vi "Express Waveform Components.vi"(8 "error in (no error)":errorcluster, 11 "Waveform":waveform(dbl)) -> (0 "error out":errorcluster, 1 "Express Waveform Attributes":T1 {"Timestamp" format="%<%X\n%x>T"; "Start Timestamp" format="%<%X\n%x>T"}, 2 "Signal Components":cluster{"X0":dbl, "dX":dbl, "Y":dbl[]} {"Y" format="%0.2f"; "dX" format="%0.6f"; "X0" format="%0.6f"}, 3 "Waveform":waveform(dbl))   [LabVIEW 2020]
uses:
  <vilib>/express/express shared/transition.llb/ex_WaveformAttribs.ctl
panel:
  in  "signal":cluster{"X0":dbl, "dX":dbl, "Y":dbl[]} {"X0" format="%.6f"; "dX" format="%.6f"; "Y" format="%0.2p"}
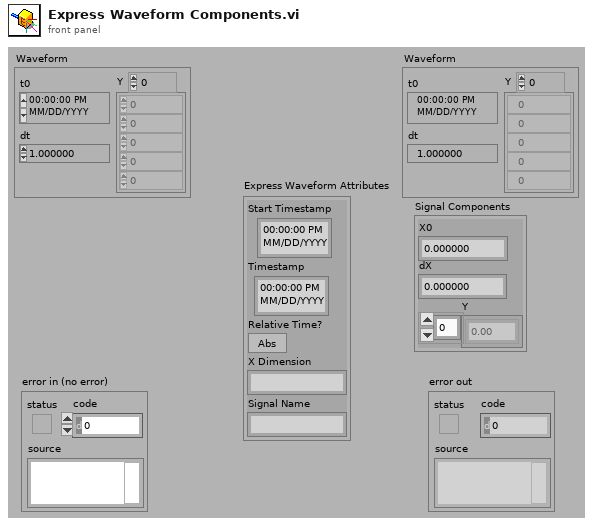
[diagram p1: front panel]
types:
  T1 = typedef "ex_WaveformAttribs.ctl" = cluster{"Start Timestamp":timestamp, "Timestamp":timestamp, "Relative Time?":bool, "X Dimension":string, "Signal Name":string}
  T2 = cluster{"Start Timestamp":timestamp, "Timestamp":timestamp, "Relative Time?":bool, "X Dimension":string, "Signal Name":string}[]
  T3 = cluster{"Start Timestamp":timestamp, "Timestamp":timestamp, "Relative Time?":bool, "X Dimension":string, "Signal Name":string}
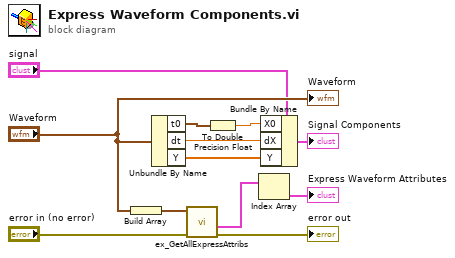
[diagram p0: block diagram]
diagram:
  n1 = Build Array("Waveform") -> (w6:waveform(dbl)[])
  n2 = Unbundle By Name("Waveform") -> ("t0"=w1:timestamp, "dt"=w9:dbl, "Y"=w8:dbl[])
  n3 = call <vilib>:"ex_GetAllExpressAttribs.vi"("error in"="error in (no error)", "Signals"=w6) -> ("error out"=→"error out":errorcluster, "All Express Wave Attributes"=w3:T2)  [unwired: 8 in]
  n4 = To Double Precision Float(number=w1) -> (double precision float=w10:dbl)
  n5 = Index Array(array=w3) -> (element=→"Express Waveform Attributes":T3)  [unwired: 1 in]
  n6 = Bundle By Name(cluster="signal", "X0"=w10, "dX"=w9, "Y"=w8) -> (→"Signal Components":cluster{"X0":dbl, "dX":dbl, "Y":dbl[]})
  "Waveform" <- "Waveform"
